vi "Populate Attr Priv.vi"(0 "TreeControl in":refnum<vi>, 2 "Data Types Dict":variant, 5 "Unique ID":string, 7 "Attribute Names":string[](array[string]), 9 "Attribute Values":variant[](array[variant]), 11 "error in":errorcluster) -> (4 "TreeControl out":refnum<vi>, 15 "error out":errorcluster)   [LabVIEW 2016, in "Tree Manager.lvclass"]
uses:
  Tree Manager.lvclass
  Tree Data/Tree Data.lvclass
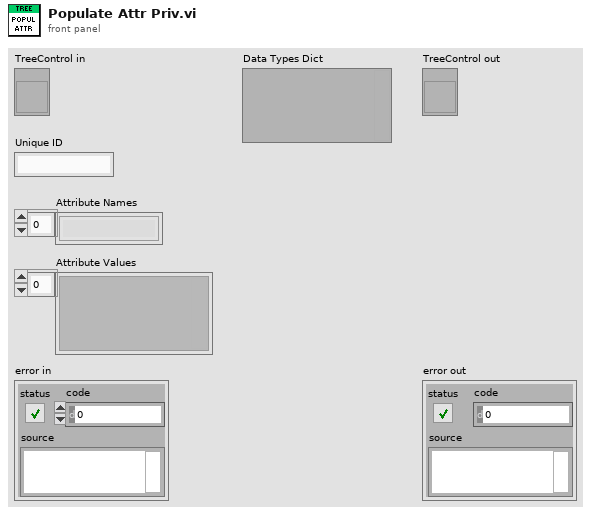
[diagram p1: front panel]
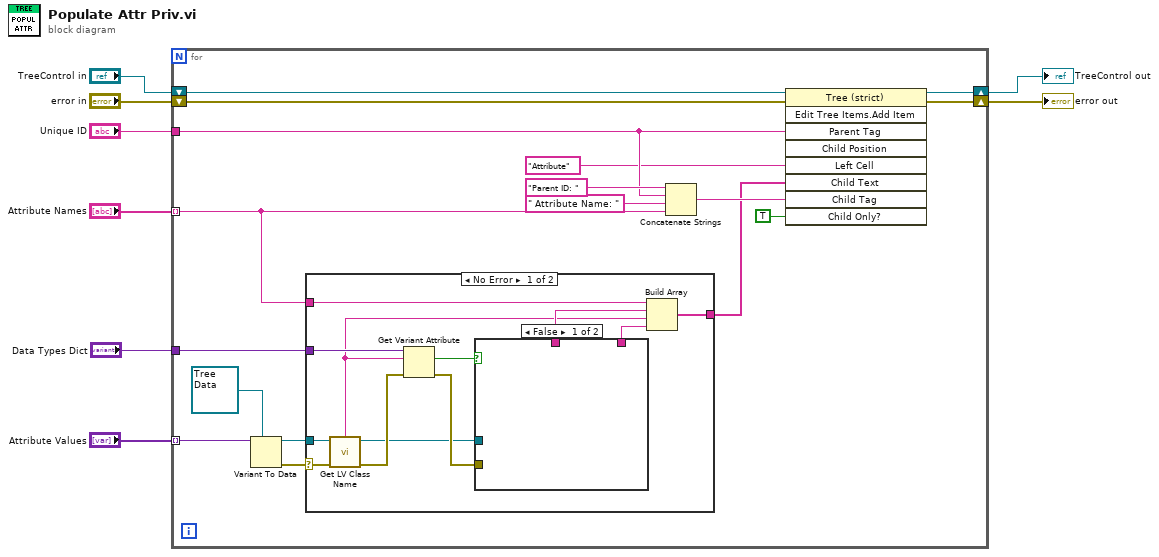
[diagram p0: block diagram]
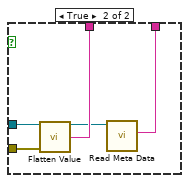
[diagram p2: hidden frame]
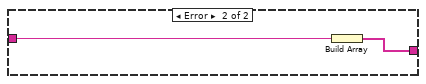
[diagram p3: hidden frame]
diagram:
  n1 = for {
    shift-right: [w22] -> w8
    shift-left: "TreeControl in" -> [w25]
    shift-right: [w21] -> w7
    shift-left: "error in" -> [w24]
    tunnel: "Attribute Names" -> [w11] mode=indexing
    tunnel: "Unique ID" -> [w18]
    tunnel: "Attribute Values" -> [w15] mode=indexing
    tunnel: "Data Types Dict" -> [w10]
    n2 = Variant To Data(type=refnum<class "Tree Data.lvclass"> refnum ("Tree Data.lvclass"), Variant=w15) -> (data=w14:refnum<class "Tree Data.lvclass">, error out=w13:errorcluster)  [unwired: 1 in]
    n3 = case shown="No Error" w13 {
      selector: w13 -> [w32 _]
      tunnel: w14 -> [w26 _]
      tunnel: [w34 w42] -> w12
      tunnel: w11 -> [w33 w43]
      tunnel: w10 -> [w31 _]
      frame No Error {
        n4 = call <vilib>:"Get LV Class Name.vi"("error in (no error)"=w32, "object"=w26) -> ("error out"=w30:errorcluster, "class name"=w27:string)  [unwired: 8 in]
        n5 = Get Variant Attribute(Variant=w31, name=w27, error in=w30) -> (found=w28:bool, error out=w29:errorcluster)  [unwired: 1 in, 2 out]
        n6 = case shown="False" w28 {
          tunnel: [_ w41] -> w36
          tunnel: [_ w40] -> w35
          tunnel: w29 -> [_ w37]
          tunnel: w26 -> [_ w38]
          frame False {
          }
          frame True {
            n7 = call-dynamic "Flatten Value.vi"("Tree Data In"=w38, "Error In"=w37) -> ("Tree Data Out"=w39:refnum<class "Tree Data.lvclass">, "Value"=w41:string)  [unwired: 11 in, 1 out]
            n8 = call "Read Meta Data.vi"("Tree Data In"=w39) -> ("Meta Data"=w40:string)  [unwired: 9 in, 1 out]
          }
        }
        n9 = Build Array(w33, w36, w27, w35) -> (w34:string[])
      }
      frame Error {
        n10 = Build Array(w43) -> (w42:string[])
      }
    }
    n11 = Concatenate Strings("Parent ID: " ("string"), w18, " Attribute Name: " ("string"), w11) -> (w17:string)
    n12 = invoke class="Tree (strict)" method="Edit Tree Items.Add Item"(reference=w25, error in=w24, "Parent Tag"=w18, "Left Cell"="Attribute" ("Left Cell String"), "Child Text"=w12, "Child Tag"=w17, "Child Only?"=TRUE) -> (reference out=w22:refnum<vi>, error out=w21:errorcluster)  [unwired: 2 in, 7 out]
  }
  "TreeControl out" <- w8
  "error out" <- w7
